vi "Gunsim Update Position.vi"(1 "cluster in":T1) -> (0 "cluster out":T1)   [LabVIEW 2015]
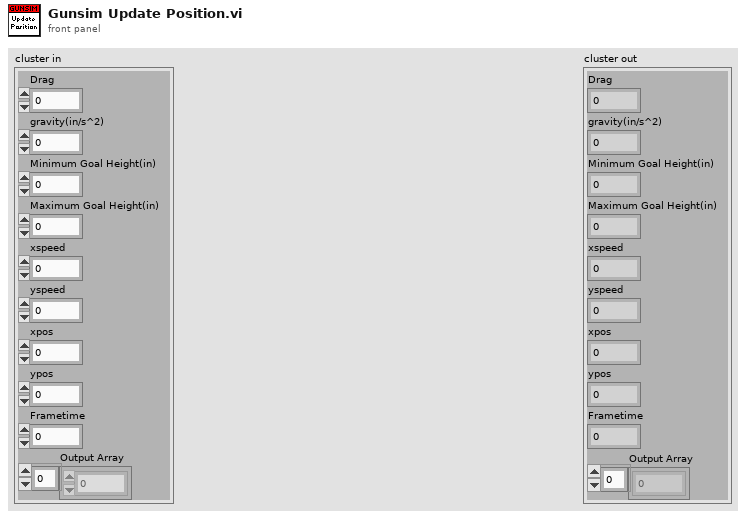
[diagram p1: front panel]
types:
  T1 = cluster{"Drag":dbl, "gravity(in/s^2)":dbl, "Minimum Goal Height(in)":dbl, "Maximum Goal Height(in)":dbl, "xspeed":dbl, "yspeed":dbl, "xpos":dbl, "ypos":dbl, "Frametime":dbl, "Output Array":dbl[]}
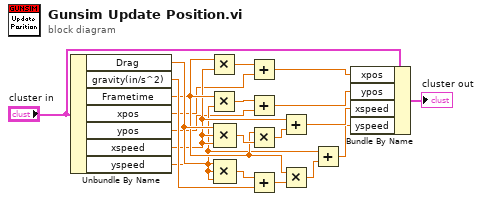
[diagram p0: block diagram]
diagram:
  n1 = Unbundle By Name("cluster in") -> ("Drag"=w12:dbl, "gravity(in/s^2)"=w13:dbl, "Frametime"=w11:dbl, "xpos"=w5:dbl, "ypos"=w3:dbl, "xspeed"=w10:dbl, "yspeed"=w4:dbl)
  n2 = Multiply(x=w11, y=w10) -> (x*y=w15:dbl)
  n3 = Multiply(x=w11, y=w4) -> (x*y=w14:dbl)
  n4 = Compound Arithmetic op=MULTIPLY(w12, w10, w10) -> (w17:dbl)
  n5 = Compound Arithmetic op=MULTIPLY(w12, w4, w4) -> (w20:dbl)
  n6 = Add(x=w15, y=w5) -> (x+y=w7:dbl)
  n7 = Add(x=w14, y=w3) -> (x+y=w8:dbl)
  n8 = Multiply(x=w11, y=w17) -> (x*y=w16:dbl)
  n9 = Add(x=w20, y=w13) -> (x+y=w19:dbl)
  n10 = Add(x=w10, y=w16) -> (x+y=w9:dbl)
  n11 = Multiply(x=w11, y=w19) -> (x*y=w18:dbl)
  n12 = Add(x=w4, y=w18) -> (x+y=w6:dbl)
  n13 = Bundle By Name(cluster="cluster in", "xpos"=w7, "ypos"=w8, "xspeed"=w9, "yspeed"=w6) -> (→"cluster out":T1)
